vi "MIN-SP-AddResultChannel.vi"(8 "Error In":errorcluster, 10 "CD Settings":T1={"CD Task Dependency"=18446744073709551615, "CD Task Dependency Ref"=18446744073709551615, "CD Task Available Wfms"=[], "CD Task Selected Wfms"=[], "Buffer Length (samples)"=0, "Min Enabled"=FALSE, "Max Enabled "=FALSE, "SP Enabled"=FALSE, "RMS Enabled"=FALSE, "Buffer Length (s)"=0.0, "Task Rate"=0.0, "Number of DAQ Chanels"=0} {"CD Task Dependency Ref" format="%.0x"; "CD Task Dependency" format="%.0x"}, 11 "Device Ref in":T2 format="%.0x") -> (0 "Error Out":errorcluster, 3 "Device Ref Out":T2=18446744073709551615 format="%.0x")   [LabVIEW 2017, in "Waveform-Processing-Custom-Device Shared.lvlib" / "Min_SP.lvlib"]
doc: "This application Adds all of the Child \"Minimum\" output channels found when the \"Add\" option is selected"
uses:
  Min_SP.lvlib
  <vilib>/NI Veristand/Custom Device API/Custom Device Item Ref.ctl
  Custom Device Settings.ctl
  <vilib>/NI Veristand/Custom Device API/Custom Device Channel.ctl
  <vilib>/NI Veristand/Custom Device API/Custom Device Channel Type.ctl
  NationalInstruments.VeriStand.SystemStorage
  Constants.vi
  <vilib>/NI Veristand/Custom Device API/Get Item Property (Dependent Node Pointer).vi
  <vilib>/NI Veristand/Custom Device API/Set Item Property (Dependent Node Pointer).vi
  System Explorer/Waveform-Processing-Custom-Device System Explorer.lvlib
  Waveform-Processing-Custom-Device Shared.lvlib
  <vilib>/NI Veristand/Custom Device API/Custom Device API.lvlib
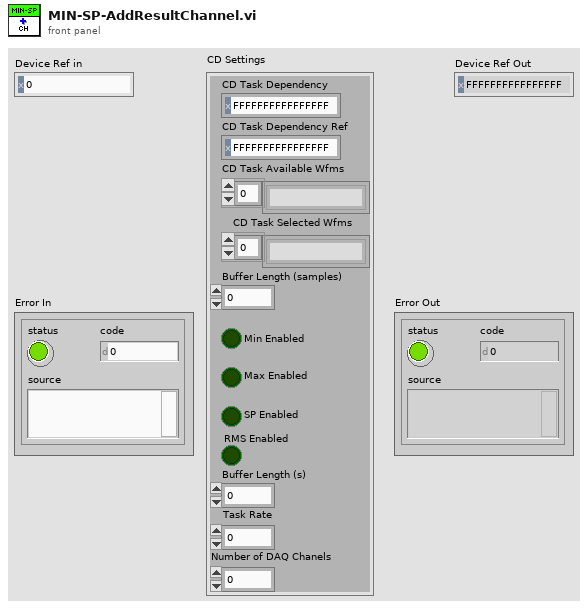
[diagram p1: front panel]
types:
  T1 = typedef "Waveform-Processing-Custom-Device Shared.lvlib/Custom Device Settings.ctl" = cluster{"CD Task Dependency":T2, "CD Task Dependency Ref":T2, "CD Task Available Wfms":string[], "CD Task Selected Wfms":string[], "Buffer Length (samples)":u32, "Min Enabled":bool, "Max Enabled ":bool, "SP Enabled":bool, "RMS Enabled":bool, "Buffer Length (s)":dbl, "Task Rate":dbl, "Number of DAQ Chanels":u32}
  T2 = typedef "Custom Device API.lvlib/Custom Device Item Ref.ctl" = u64
  T3 = typedef "Custom Device API.lvlib/Custom Device Channel Type.ctl" = enum16{"Input", "Output"}
  T4 = typedef "Custom Device API.lvlib/Custom Device Channel.ctl" = cluster{"Type":T3, "Units":string, "Default Value":dbl, "Faultable":bool, "Scalable":bool}
  T5 = cluster{"Waveform Name":string, "Units":string}[]
  T6 = typedef "Custom Device API.lvlib/Custom Device Pointer.ctl" = refnum<k24>
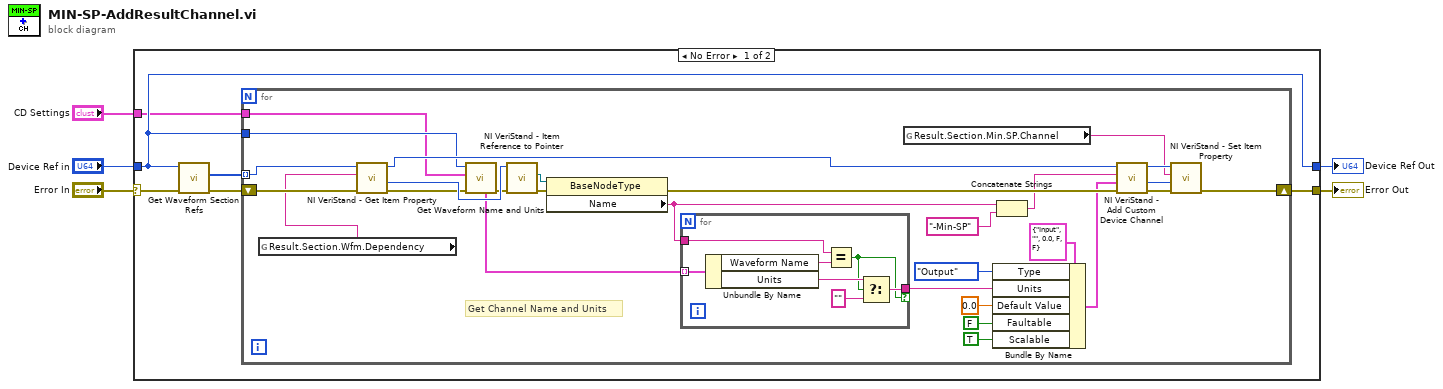
[diagram p0: block diagram]
diagram:
  n1 = case shown="No Error" "Error In" {
    selector: "Error In" -> [w11 w48]
    tunnel: [w8 w48] -> w5
    tunnel: "Device Ref in" -> [w7 w47]
    tunnel: [w7 w47] -> w2
    tunnel: "CD Settings" -> [w6 _]
    frame No Error {
      n2 = call "Get Waveform Section Refs.vi"("Error in"=w11, "Device Ref in"=w7) -> ("Error out"=w10:errorcluster, "Result Section Refs"=w9:T2[])  [unwired: 7 in, 1 out]
      n3 = for {
        tunnel: w9 -> [w38] mode=indexing
        shift-right: [w29] -> w8
        shift-left: w10 -> [w39]
        tunnel: w7 -> [w16]
        tunnel: w6 -> [w15]
        # "Get Channel Name and Units"
        n4 = global read "Constants.vi" "Result.Section.Wfm.Dependency"() -> (w25:string)
        n5 = call-poly <vilib>:"NI VeriStand - Get Item Property.vi"("error in (no error)"=w39, "Property Name"=w25, "Item Ref in"=w38) -> ("error out"=w24:errorcluster, "Dependent Node Ref"=w37:T2, "Item Ref out"=w31:T2)  [unwired: 5 in, 1 out]
        n6 = call "Get Waveform Name and Units.vi"("Error In"=w24, "CD Settings"=w15, "CustomDevice Ref"=w16) -> ("Error Out"=w23:errorcluster, "Waveform Channel Name and Units"=w17:T5)  [unwired: 7 in]
        n7 = call <vilib>:"NI VeriStand - Item Reference to Pointer.vi"("error in (no error)"=w23, "Item Ref in"=w37) -> ("error out"=w36:errorcluster, "Node Pointer"=w35:T6)  [unwired: 6 in, 2 out]
        n8 = property class="BaseNodeType"(reference=w35, error in=w36) -> (error out=w33:errorcluster, "Name"=w14:string)  [unwired: 1 out]
        n9 = for {
          tunnel: w17 -> [w45] mode=indexing
          tunnel: w14 -> [w46]
          tunnel: [w42] -> w18 if=w40
          n10 = Unbundle By Name(w45) -> ("Waveform Name"=w44:string, "Units"=w43:string)
          n11 = Equal?(x=w46, y=w44) -> (x = y?=w40:bool)
          n12 = Select(t=w43, s=w40, f="") -> (s? t:f=w42:string)
        }
        n13 = global read "Constants.vi" "Result.Section.Min.SP.Channel"() -> (w27:string)
        n14 = Bundle By Name(cluster=T4 {"Type"=enum."Input", "Units"="", "Default Value"=0.0, "Faultable"=FALSE, "Scalable"=FALSE} ("Channel"), "Type"=Custom_Device_Channel_Type."Output", "Units"=w18, "Default Value"=0.0, "Faultable"=FALSE, "Scalable"=TRUE) -> (w12:T4)
        n15 = Concatenate Strings(w14, "-Min-SP" ("Property Name")) -> (w32:string)
        n16 = call <vilib>:"NI VeriStand - Add Custom Device Channel.vi"("error in (no error)"=w33, "Channel"=w12, "Channel Name"=w32, "Parent Ref in"=w31) -> ("error out"=w30:errorcluster, "Channel Ref"=w26:T2, "Parent Ref out"=w28:T2)  [unwired: 4 in, 1 out]
        n17 = call-poly <vilib>:"NI VeriStand - Set Item Property.vi"("error in (no error)"=w30, "Dependent Node Ref"=w26, "Property Name"=w27, "Item Ref in"=w28) -> ("error out"=w29:errorcluster)  [unwired: 5 in, 2 out]
      }
    }
    frame Error {
    }
  }
  "Error Out" <- w5
  "Device Ref Out" <- w2
